vi "Transfer_Curve.vi"(0 "File Path":path=path "C:/DATA/raj/transferdump.txt.txt", 1 "V_G Start":dbl=-0.7 format="%#.3g", 3 "V_G Finish":dbl=0.4 format="%#.3g", 4 "V_G Step Size":dbl=0.05 format="%#.3g", 5 "Preread delay (ms)":dbl=10000.0 format="%.2f", 7 "Delay between \naverages (ms)":dbl=200.0 format="%#.3f", 8 "Keithley 237 GPIB address":string="17", 9 "Software Averages":i16=5, 12 "VISA resource name":refnum<visa-resource-name>="GPIB0::24::INSTR", 13 "First bias settle (ms)":dbl=60000.0 format="%#.2f", 15 "Current Compliance\nLimit (A) Ke2400":dbl=1.0 format="%#.3e", 18 "Dimensions":T1(ring), 24 "Voltage Compliance Limit 237 (V)":dbl=10.0 format="%#.3f", 25 "Current Compliance\nLimit 237 (A)":dbl=0.1 format="%#.3f", 27 "V_DS":dbl=-0.6 format="%#_13g") -> ()   [LabVIEW 2018]
uses:
  <vilib>/Utility/file.llb/Write Delimited Spreadsheet (string).vi
  Instance           1 16Saved   JV curve .vi
  <userlib>/KE237.LLB/Keith 237 Operate/Standby.vi
  <instrlib>/Keithley 24XX/Public/Data/Read (Single Point).vi
  <vilib>/Analysis/NI_AALBase.lvlib
  <instrlib>/Keithley 24XX/Keithley 24XX.lvlib
panel:
  in  "Quick Burn In?":bool
  out "timer":dbl format="%#_6f"
  out "Keithley 2400":cluster{dbl[], dbl[]}(graph)={[-2.0, -1.9, -1.8, -1.7, -1.6, -1.5], [-6.6965744e-11, -6.7804984e-11, -6.685451799999999e-11, -6.6450076e-11, -6.5125542e-11, -6.7339852e-11]}
  out "I_G (A)":dbl=-6.642986e-11 format="%.2e"
  in  "Autozero?":u16(ring) items=["On", "Off", "Once"]
  in  "Measurement Speed (1 PLC)":dbl=1.0 format="%.2g"
  in  "Manual Range (Max I)":dbl=1.0
  in  "Enable Meas Auto Range":bool=TRUE
  in  "Source Mode":u16(ring) items=["Voltage", "Current"]
  in  "Return Sweep?":bool=TRUE
  out "I_DS":dbl=-1.38e-12 format="%.2e"
  out "Outputfile":path=path "C:/DATA/Mark Ziffer/test10"
  in  "Abort Scan":bool=TRUE
  out "V_G":dbl=-1.5 format="%#.2f"
  out "Keithley 237":cluster{dbl[], dbl[]}(graph)={[-2.0, -1.9, -1.8, -1.7, -1.6, -1.5], [-6.720000000000001e-13, -2.18e-13, -2.7599999999999993e-13, -8.999999999999998e-14, -1.3999999999999998e-13, -1.3800000000000002e-13]}
  # "Transfer Curve\nbased on  EL_photocurrent_JV.vi for controlling 2 Ketthleys\n\n9/2017 MZ"
  # "Software Settings"
  # "Ke237 Settings"
  # "Ke2400 Settings"
  # "Notes for IV Scan\n\n2010.07.06 - add absolute value plotter to look at log-scale current\n2010.01.07 - Modified file headers for distinguihing when imported to Igor Pro - the prefix of each header will be the file name.\n2009.01.15 - I updated the code to run on the VISA driver convention. I also modified the file saving and the option to set the\n                      graph display.\n2008.12.01 - I fixed an issue with calculations of J. It was mis-wired to divide current by wavelength, rather than active area.  BM\n\n=========================\nI added the functionality to calculate the fill factor, rectification ratio, short circuit current density, and open circuit voltage. \nAdditionally, current density (mA/cm^2) is reported in the plot window and column B of the data file, and the current (A) has been \nmoved to column C. Open circuit voltage is linearly interpolated. The max power point (mpp) for calculating fill factor is taken as \nthe data point with the highest I-V product, so this makes it only as accurate as your voltage step size, but should be fine for a decent \ndevice on the 50 mV default step size.\n\nIf you know how to use the previous versions of IV scan, \nmake sure you set these parameters before you scan:\n1) Recftification Ratio Bias - this is the +/- bias value you wish to record a rectification ratio at.\n2) Effective Area - this is the area in cm^2 of the diode mask (photoactive area) when measuring under illumination or the measured \n     area of the electrode overlap when measured in dark (regular active area).\n3) Do you want to record a separate data file for the calculated characteristics? If so, make sure the switch is on.\n\nAs of today, I couldn't figure out how to append the computed characteristics to the I-V file without experiencing formating issues, so\nI opted to just create a separate file if you want to save that info. Feel free to fix this if you know how. Check tab 3 > tab 2 > tab 9 in the\nblock diagram.\n\n2008-04-15\nB MacLeod"
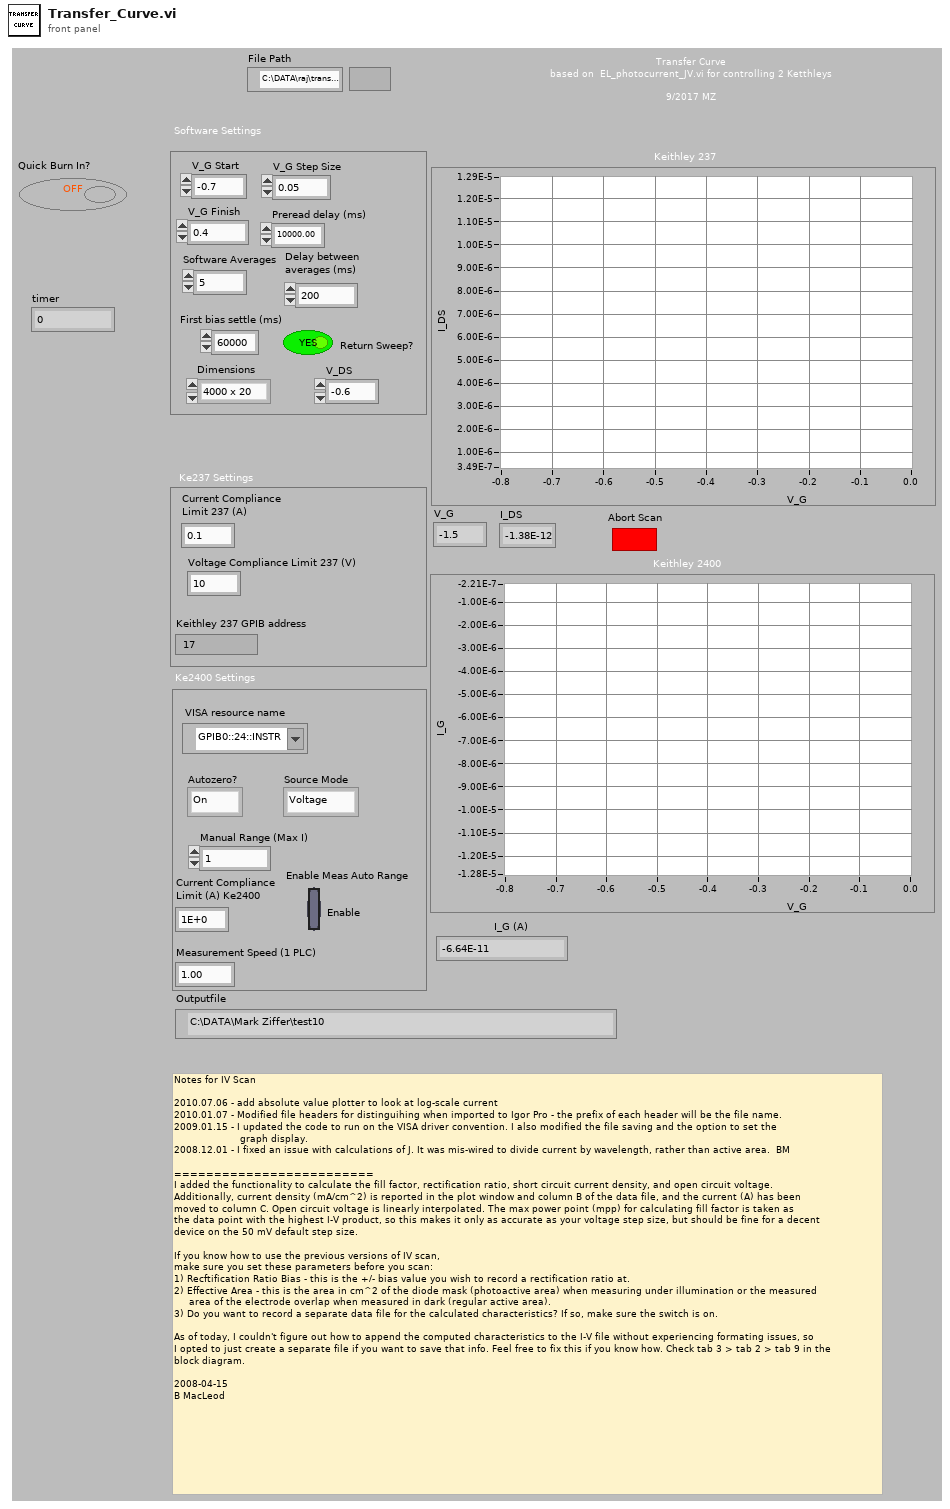
[diagram p1: front panel]
types:
  T1 = enum16{"4000 x 20", "2000 x 20", "1000 x 20", "800 x 20", "400 x 20", "200 x 20", "100 x 20"}
  T2 = cluster{"error":bool, "code":i32, "source":string}
  T3 = cluster{"source value":string, "measure value":string, "delay value (sec)":string, "time value (sec)":string}[]
  T4 = cluster{"source value":dbl, "measure value":dbl, "delay value (sec)":dbl, "time value (sec)":dbl}[]
  T5 = cluster{"[0]":cluster{"source value":dbl, "measure value":dbl, "delay value (sec)":dbl, "time value (sec)":dbl}, "[1]":cluster{"source value":dbl, "measure value":dbl, "delay value (sec)":dbl, "time value (sec)":dbl}, "[2]":cluster{"source value":dbl, "measure value":dbl, "delay value (sec)":dbl, "time value (sec)":dbl}, "[3]":cluster{"source value":dbl, "measure value":dbl, "delay value (sec)":dbl, "time value (sec)":dbl}, "[4]":cluster{"source value":dbl, "measure value":dbl, "delay value (sec)":dbl, "time value (sec)":dbl}, "[5]":cluster{"source value":dbl, "measure value":dbl, "delay value (sec)":dbl, "time value (sec)":dbl}, "[6]":cluster{"source value":dbl, "measure value":dbl, "delay value (sec)":dbl, "time value (sec)":dbl}, "[7]":cluster{"source value":dbl, "measure value":dbl, "delay value (sec)":dbl, "time value (sec)":dbl}, "[8]":cluster{"source value":dbl, "measure value":dbl, "delay value (sec)":dbl, "time value (sec)":dbl}}
  T6 = cluster{"source value":dbl, "measure value":dbl, "delay value (sec)":dbl, "time value (sec)":dbl}
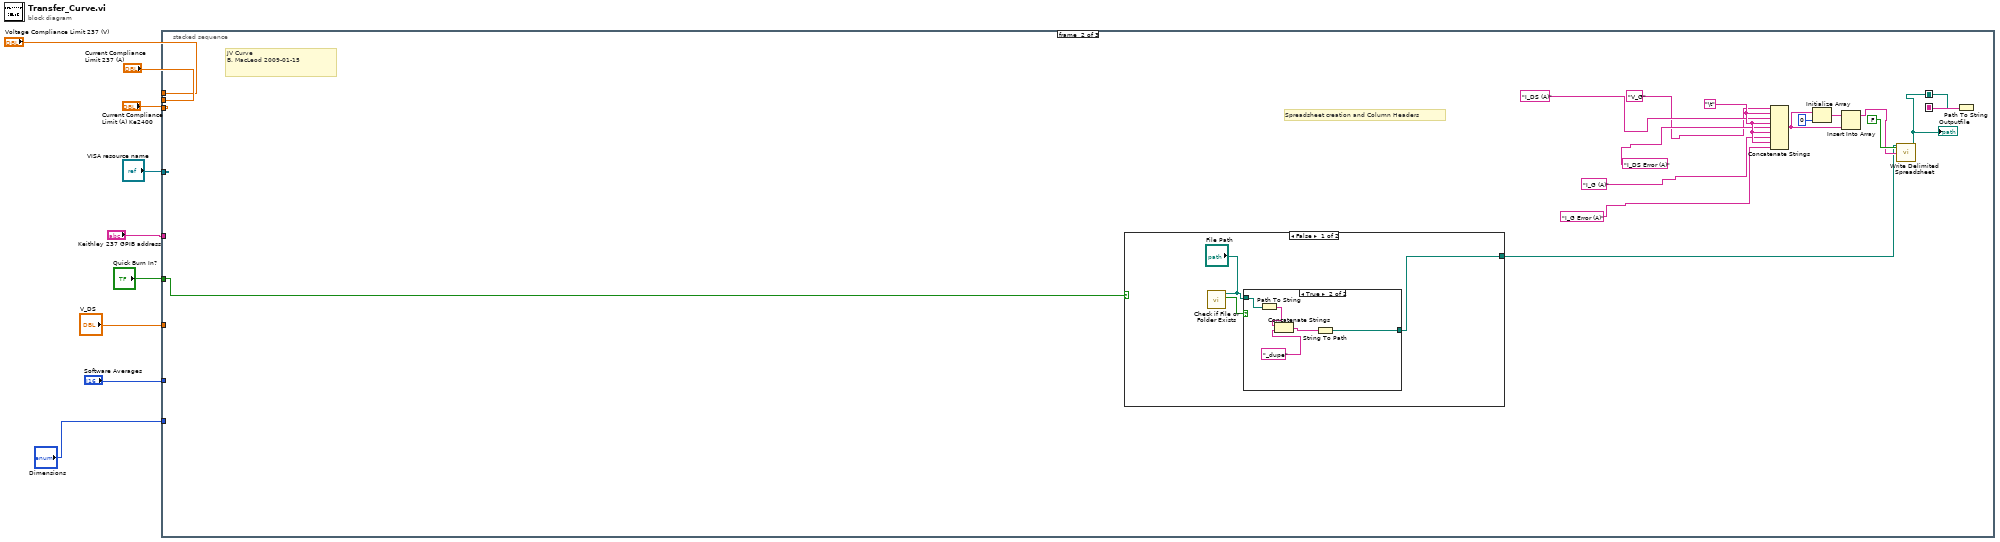
[diagram p0: block diagram]
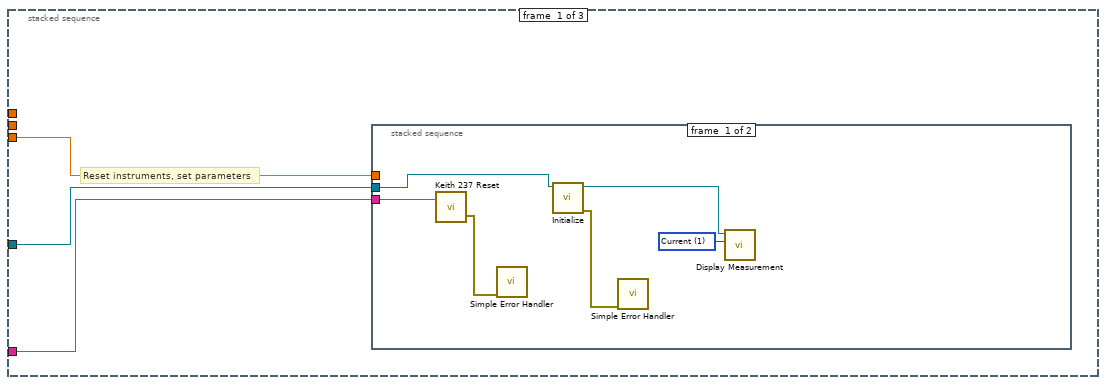
[diagram p2: hidden frame]
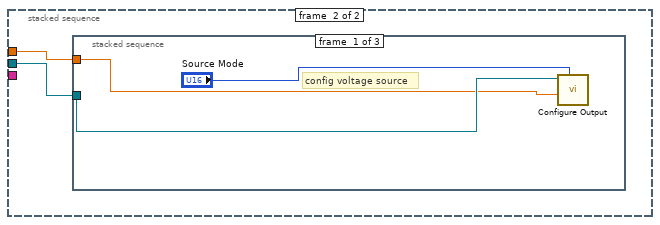
[diagram p3: hidden frame]
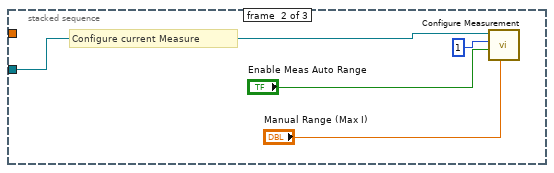
[diagram p4: hidden frame]
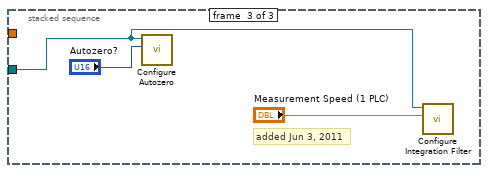
[diagram p5: hidden frame]
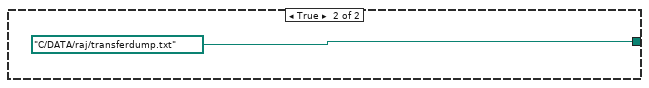
[diagram p7: hidden frame]
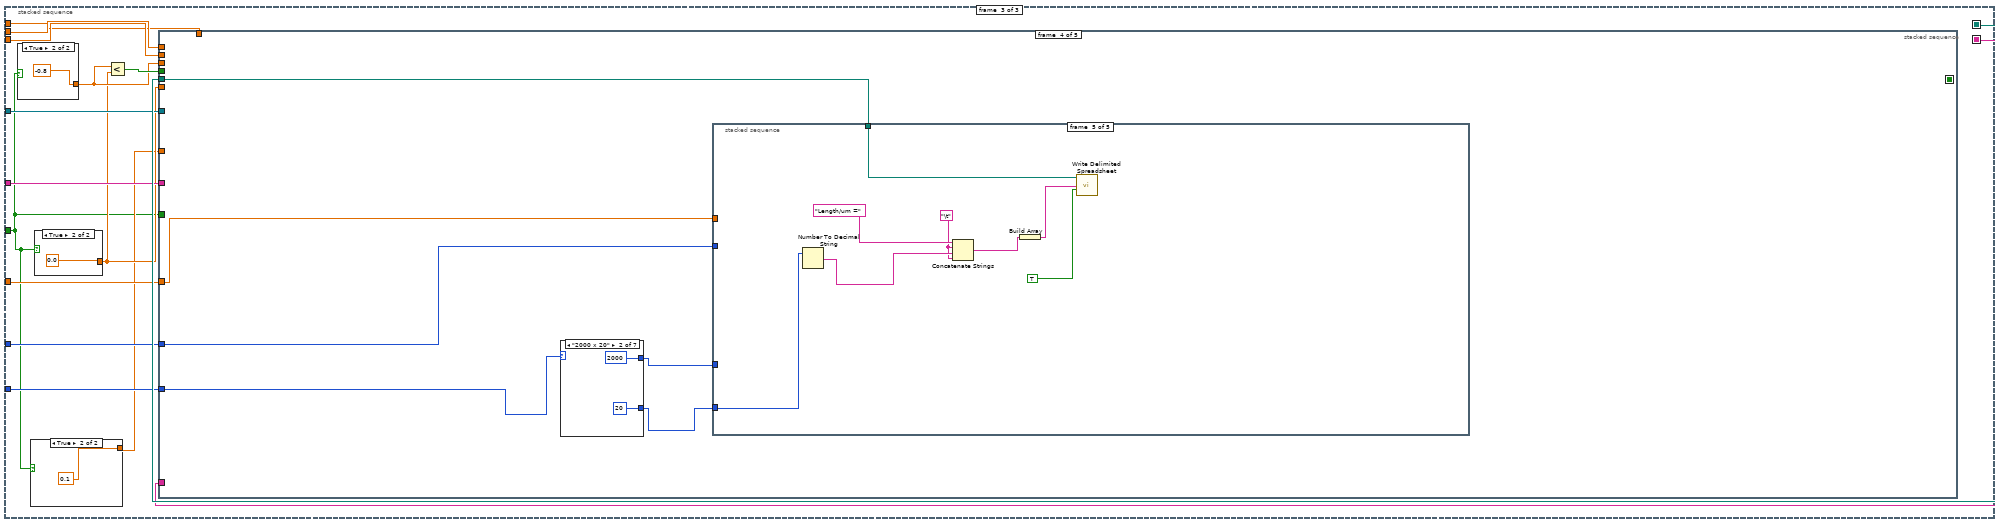
[diagram p8: hidden frame]
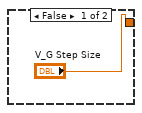
[diagram p9: hidden frame]
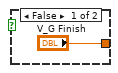
[diagram p10: hidden frame]
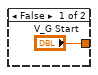
[diagram p11: hidden frame]
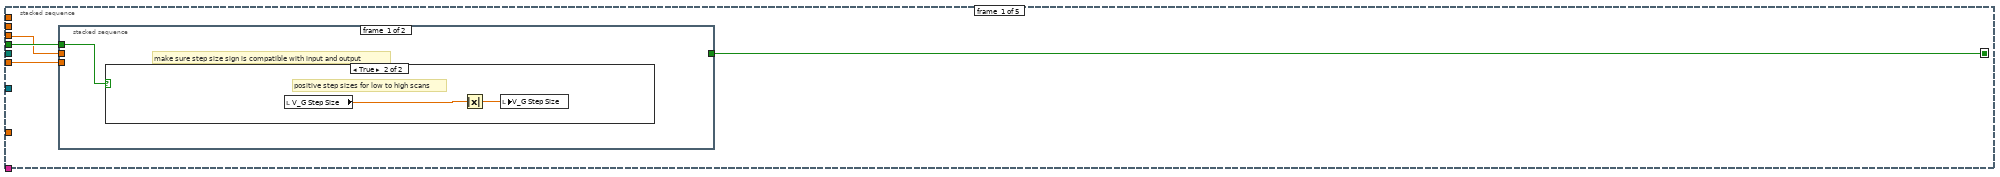
[diagram p12: hidden frame]
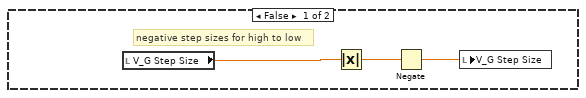
[diagram p13: hidden frame]
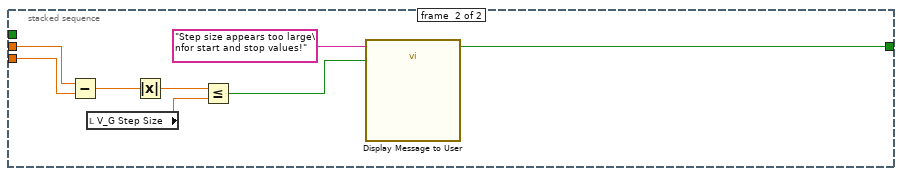
[diagram p14: hidden frame]
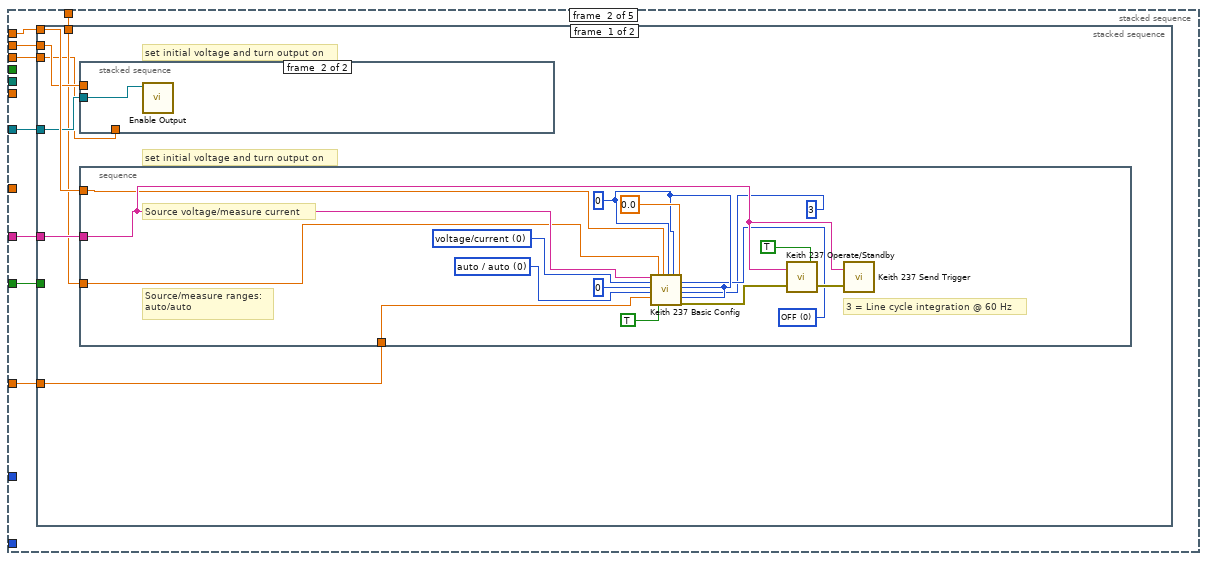
[diagram p15: hidden frame]
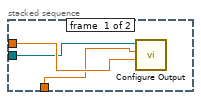
[diagram p16: hidden frame]
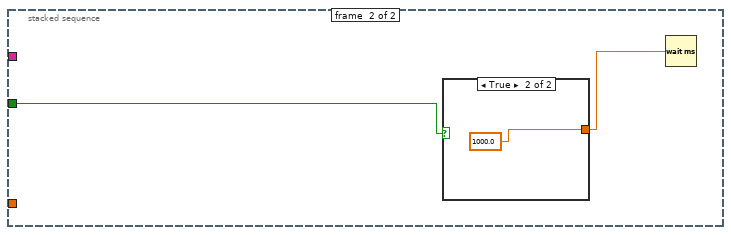
[diagram p17: hidden frame]
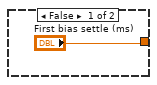
[diagram p18: hidden frame]
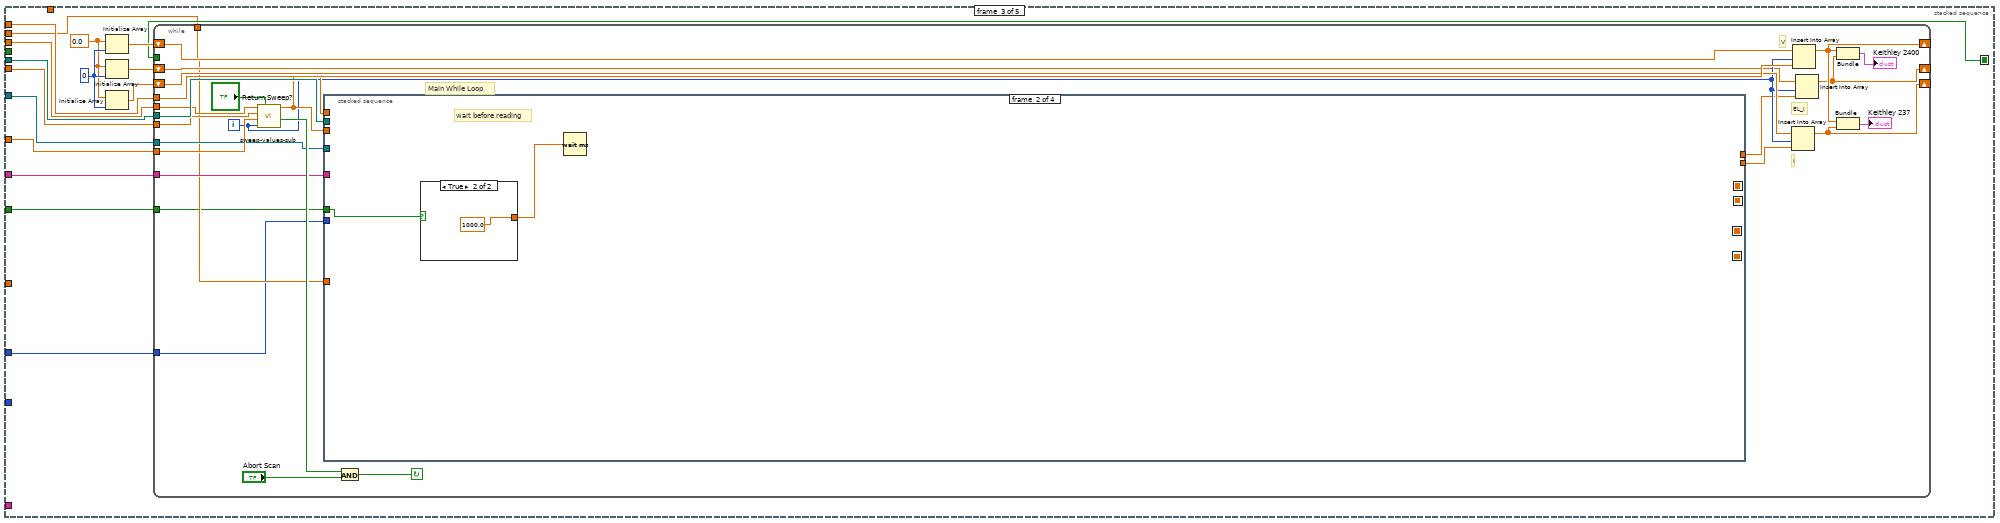
[diagram p19: hidden frame]
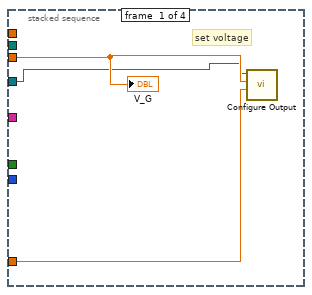
[diagram p20: hidden frame]
diagram:
  # "JV Curve\nB. MacLeod 2009-01-15"
  n1 = stacked-sequence {
    seq-local: [_ w38 _] -> [_ _ w69]
    seq-local: [_ w45 _] -> [_ _ w68]
    tunnel: "Current Compliance\nLimit 237 (A)" -> [_ _ w67]
    tunnel: "Voltage Compliance Limit 237 (V)" -> [_ _ w63]
    tunnel: "Keithley 237 GPIB address" -> [w12 _ w66]
    tunnel: "VISA resource name" -> [w11 _ w65]
    tunnel: "Current Compliance\nLimit (A) Ke2400" -> [w10 _ w64]
    tunnel: "V_DS" -> [_ _ w62]
    tunnel: "Software Averages" -> [_ _ w61]
    tunnel: "Dimensions" -> [_ _ w60]
    tunnel: "Quick Burn In?" -> [_ w31 w56]
    frame #0 {
      # "Reset instruments, set parameters"
      n2 = stacked-sequence {
        tunnel: w12 -> [w17 _]
        tunnel: w11 -> [w16 w20]
        tunnel: w10 -> [_ w19]
        frame #0 {
          w15 = u16 1 items=["Voltage", "Current", "Resistance"] ("Displayed Measurement (0: Voltage)")
          n3 = call <userlib>:"Keith 237 Reset.vi"("GPIB address"=w17) -> ("error out"=w18:T2)  [unwired: 1 in]
          n4 = call <vilib>:"Simple Error Handler.vi"("error in (no error)"=w18) -> ()  [unwired: 1 in, 8 out]
          n5 = call <instrlib>:"Initialize.vi"("VISA resource name"=w16) -> ("error out"=w13:errorcluster, "VISA resource name out"=w14:refnum<visa-resource-name>)  [unwired: 9 in]
          n6 = call <vilib>:"Simple Error Handler.vi"("error in (no error)"=w13) -> ()  [unwired: 1 in, 8 out]
          n7 = call <instrlib>:"Display Measurement.vi"("Displayed Measurement (0: Voltage)"=w15, "VISA resource name"=w14) -> ()  [unwired: 8 in, 2 out]
        }
        frame #1 {
          n8 = stacked-sequence {
            tunnel: w20 -> [w22 w24 w28]
            tunnel: w19 -> [w21 _ _]
            frame #0 {
              # "config voltage source"
              n9 = call <instrlib>:"Configure Output.vi"("Source Mode  (0: Voltage)"="Source Mode", "Compliance  Level (0.1)"=w21, "VISA resource name"=w22) -> ()  [unwired: 3 in, 6 out]
            }
            frame #1 {
              # "Configure current Measure"
              n10 = call <instrlib>:"Configure Measurement.vi"("Manual Range (1.0)"="Manual Range (Max I)", "Enable Auto Range (T:Enable)"="Enable Meas Auto Range", "Function (0: Volts)"=1, "VISA resource name"=w24) -> ()  [unwired: 1 in, 7 out]
            }
            frame #2 {
              # "added Jun 3, 2011"
              n11 = call <instrlib>:"Configure Autozero.vi"("Autozero  (0: On)"="Autozero?", "VISA resource name"=w28) -> ()  [unwired: 1 in, 9 out]
              n12 = call <instrlib>:"Configure Integration Filter.vi"("Measurement Speed (1 PLC)"="Measurement Speed (1 PLC)", "VISA resource name"=w28) -> ()  [unwired: 8 in, 2 out]
            }
          }
        }
      }
    }
    frame #1 {
      w41 = "\t"
      # "Spreadsheet creation and Column Headers"
      n13 = case shown="False" w31 {
        tunnel: [w46 path "C:/DATA/raj/transferdump.txt"] -> w32
        frame False {
          n14 = call <vilib>:"Check if File or Folder Exists.vi"("path"="File Path") -> ("file or folder exists?"=w48:bool)  [unwired: 8 in, 2 out]
          n15 = case shown="True" w48 {
            tunnel: "File Path" -> [w49 w53]
            tunnel: [w49 w50] -> w46
            frame False {
            }
            frame True {
              n16 = Path To String(path=w53) -> (string=w54:string)
              n17 = Concatenate Strings(w54, "_dupe") -> (w51:string)
              n18 = String To Path(string=w51) -> (path=w50:path)
            }
          }
        }
        frame True {
        }
      }
      n19 = Concatenate Strings("V_G", w41, "I_DS (A)", w41, "I_DS Error (A)", w41, "I_G (A)", w41, "I_G Error (A)" ("string")) -> (w43:string)
      n20 = Initialize Array(w43, 0 ("dimension size")) -> (w42:string[])
      n21 = Insert Into Array(array=w42, new element=w43) -> (w39:string[])  [unwired: 1 in]
      n22 = call-poly <vilib>:"Write Delimited Spreadsheet.vi"("file path (dialog if empty)"=w32, "1D data"=w39, "transpose? (no:F)"=FALSE ("append to file? (new file:F)")) -> ("new file path (Not A Path if cancelled)"=w38:path)  [unwired: 11 in, 1 out]
      "Outputfile" <- w38
      n23 = Path To String(path=w38) -> (string=w45:string)
    }
    frame #2 {
      n24 = case shown="True" w56 {
        tunnel: ["V_G Start" -0.8] -> w59
        frame False {
        }
        frame True {
        }
      }
      n25 = case shown="True" w56 {
        tunnel: ["V_G Step Size" 0.1] -> w57
        frame False {
        }
        frame True {
        }
      }
      n26 = case shown="True" w56 {
        tunnel: ["V_G Finish" 0.0] -> w58
        frame False {
        }
        frame True {
        }
      }
      n27 = Less?(x=w59, y=w58) -> (x < y?=w70:bool)
      n28 = stacked-sequence {
        seq-local: [w77 _ _ _ _] -> [_ _ w141 _ _]
        tunnel: w70 -> [w80 _ _ _ _]
        tunnel: w59 -> [w79 w97 w147 _ _]
        tunnel: w58 -> [w78 _ w148 _ _]
        tunnel: w57 -> [_ _ w146 _ _]
        tunnel: w69 -> [_ _ w145 w225 _]
        tunnel: w68 -> [_ _ _ _ _]
        tunnel: w67 -> [_ w102 w142 _ _]
        tunnel: w66 -> [_ w101 w140 _ w281]
        tunnel: w65 -> [_ w99 w139 _ w280]
        tunnel: w64 -> [_ w100 w135 _ _]
        tunnel: w63 -> [_ w98 _ _ _]
        tunnel: w62 -> [_ w96 _ w226 _]
        tunnel: w61 -> [_ _ w134 w224 _]
        tunnel: w60 -> [_ _ _ w223 _]
        tunnel: w56 -> [_ w95 w133 _ _]
        frame #0 {
          n29 = stacked-sequence {
            tunnel: w80 -> [w81 _]
            tunnel: w79 -> [_ w94]
            tunnel: w78 -> [_ w93]
            tunnel: [_ w87] -> w77
            frame #0 {
              # "make sure step size sign is compatible with input and output"
              n30 = case shown="True" w81 {
                frame False {
                  # "negative step sizes for high to low"
                  n31 = local read "V_G Step Size"() -> (w84:dbl)
                  n32 = Absolute Value(x=w84) -> (abs(x)=w83:dbl)
                  n33 = Negate(x=w83) -> (-x=w82:dbl)
                  n34 = local write "V_G Step Size"(w82) -> ()
                }
                frame True {
                  # "positive step sizes for low to high scans"
                  n35 = local read "V_G Step Size"() -> (w86:dbl)
                  n36 = Absolute Value(x=w86) -> (abs(x)=w85:dbl)
                  n37 = local write "V_G Step Size"(w85) -> ()
                }
              }
            }
            frame #1 {
              n38 = Subtract(x=w94, y=w93) -> (x-y=w92:dbl)
              n39 = local read "V_G Step Size"() -> (w90:dbl)
              n40 = Absolute Value(x=w92) -> (abs(x)=w91:dbl)
              n41 = Less Or Equal?(x=w91, y=w90) -> (x <= y?=w88:bool)
              n42 = call "Display Message to User"("Enable"=w88, "Message"="Step size appears too large\nfor start and stop values!") -> ("OK"=w87:bool)  [unwired: 1 in, 8 out]
            }
          }
        }
        frame #1 {
          n43 = stacked-sequence {
            tunnel: w102 -> [w109 _]
            tunnel: w101 -> [w108 _]
            tunnel: w100 -> [w107 _]
            tunnel: w99 -> [w106 _]
            tunnel: w98 -> [w105 _]
            tunnel: w97 -> [w104 _]
            tunnel: w96 -> [w103 _]
            tunnel: w95 -> [_ w130]
            frame #0 {
              # "set initial voltage and turn output on"
              # "set initial voltage and turn output on"
              n44 = stacked-sequence {
                tunnel: w107 -> [w112 _]
                tunnel: w106 -> [w111 w113]
                tunnel: w104 -> [w110 _]
                frame #0 {
                  n45 = call <instrlib>:"Configure Output.vi"("Compliance  Level (0.1)"=w112, "Output Level (0)"=w110, "VISA resource name"=w111) -> ()  [unwired: 3 in, 6 out]
                }
                frame #1 {
                  n46 = call <instrlib>:"Enable Output.vi"("VISA resource name"=w113) -> ()  [unwired: 2 in, 9 out]
                }
              }
              n47 = stacked-sequence {
                tunnel: w109 -> [w117]
                tunnel: w108 -> [w119]
                tunnel: w105 -> [w116]
                tunnel: w103 -> [w114]
                frame #0 {
                  w118 = u16 0 items=["OFF", "ON"] ("default delay (on:1)")
                  w120 = u16 0 items=["auto / auto", "1 nA / 1.1 V", "10 nA / 11 V", "100 nA / 110 V", "0.001 mA / 1100 V", "0.01 mA / 1100 V", "0.1 mA / 1100 V", "1 mA / 1100 V", "10 mA / 1100 V", "100 mA / 1100 V"] ("source range\nI source / V source (auto:0)")
                  w121 = u16 0 items=["voltage/current", "current/voltage"] ("source/measure (V/I:0)")
                  w123 = u16 0
                  # "3 = Line cycle integration @ 60 Hz"
                  # "Source/measure ranges:\nauto/auto"
                  # "Source voltage/measure current"
                  n48 = call <userlib>:"Keith 237 Basic Config.vi"("GPIB address"=w119, "source/measure (V/I:0)"=w121, "function (DC:0)"=u16 0, "source range\nI source / V source (auto:0)"=w120, "source level"=w114, "voltage \ncompliance level"=w116, "1100 V range (disabled:F)"=TRUE, "current \ncompliance level"=w117, "compliance/\nmeasurement range (auto:0)"=w123, "suppression (off:0)"=w123, "DC delay (sec)"=0.0, "default delay (on:1)"=w118, "filter (disabled:0)"=w123, "integration time (medium:1)"=u16 3, "sense (local:0)"=w123) -> ("error out"=w128:T2)  [unwired: 4 in]
                  n49 = call "Keith 237 Operate/Standby.vi"("source"=TRUE, "error in"=w128, "GPIB address"=w119) -> ("error out"=w126:T2)
                  n50 = call <userlib>:"Keith 237 Send Trigger.vi"("GPIB address"=w119, "error in"=w126) -> ()  [unwired: 1 out]
                }
              }
            }
            frame #1 {
              n51 = case shown="True" w130 {
                tunnel: ["First bias settle (ms)" 1000.0] -> w129
                frame False {
                }
                frame True {
                }
              }
              n52 = Wait (ms)(milliseconds to wait=w129) -> ()  [unwired: 1 out]
            }
          }
        }
        frame #2 {
          w138 = 0
          w137 = 0.0
          n53 = Initialize Array(w137, w138) -> (w144:dbl[])
          n54 = Initialize Array(w137, w138) -> (w136:dbl[])
          n55 = Initialize Array(w137, w138) -> (w143:dbl[])
          n56 = while {
            shift-left: w143 -> [w170]
            shift-right: [w158] -> _
            shift-left: w144 -> [w171]
            shift-right: [w161] -> _
            tunnel: w145 -> [w173]
            tunnel: w146 -> [w169]
            tunnel: w147 -> [w168]
            tunnel: w148 -> [w167]
            tunnel: w142 -> [w165]
            tunnel: w141 -> [_]
            shift-right: [w157] -> _
            shift-left: w136 -> [w153]
            tunnel: w140 -> [w156]
            tunnel: w139 -> [w155]
            tunnel: w135 -> [w151]
            tunnel: w134 -> [w150]
            tunnel: w133 -> [w149]
            i -> [w159]
            stop <- w163 continue-if-true
            # "EL_I"
            # "Main While Loop"
            # "V"
            # "I"
            n57 = call "sweep-values-sub.vi"("Forward/Reverse"="Return Sweep?", "Point Number"=w159, "Step Size"=w169, "Sweep Stop"=w167, "Sweep Start"=w168) -> ("Active"=w164:bool, "Output"=w172:dbl)  [unwired: 2 out]
            n58 = stacked-sequence {
              seq-local: [_ _ w190 _] -> [_ _ _ w207]
              seq-local: [_ _ w184 _] -> [_ _ _ w208]
              seq-local: [_ _ w186 _] -> [_ _ _ w206]
              seq-local: [_ _ w185 _] -> [_ _ _ w205]
              tunnel: [_ _ w184 _] -> w160
              tunnel: w172 -> [w177 _ _ w219]
              tunnel: w173 -> [_ _ _ w210]
              tunnel: w165 -> [_ _ _ _]
              tunnel: w156 -> [_ _ w188 _]
              tunnel: w155 -> [w175 _ w187 _]
              tunnel: [_ _ w186 _] -> w154
              tunnel: w151 -> [w176 _ _ _]
              tunnel: w150 -> [_ _ w183 _]
              tunnel: w149 -> [_ w178 _ _]
              frame #0 {
                # "set voltage"
                n59 = call <instrlib>:"Configure Output.vi"("Compliance  Level (0.1)"=w176, "Output Level (0)"=w177, "VISA resource name"=w175) -> ()  [unwired: 3 in, 6 out]
                "V_G" <- w177
              }
              frame #1 {
                # "wait before reading"
                n60 = case shown="True" w178 {
                  tunnel: ["Preread delay (ms)" 1000.0] -> w179
                  frame False {
                  }
                  frame True {
                  }
                }
                n61 = Wait (ms)(milliseconds to wait=w179) -> ()  [unwired: 1 out]
              }
              frame #2 {
                # "I_DS"
                # "I_G"
                # "read values"
                n62 = for {
                  N: w183 -> [_]
                  tunnel: [w194] -> w189 mode=indexing
                  tunnel: w188 -> [w193]
                  tunnel: w187 -> [w192]
                  tunnel: [w191] -> w182 mode=indexing
                  n63 = stacked-sequence {
                    tunnel: [w199 _] -> w194
                    tunnel: w193 -> [w197 _]
                    tunnel: w192 -> [w196 _]
                    tunnel: [w195 _] -> w191
                    frame #0 {
                      n64 = call <userlib>:"Keith 237 Read Measurement.vi"("GPIB address"=w197) -> ("display"=w202:T3)  [unwired: 1 in, 3 out]
                      n65 = call-poly <instrlib>:"Read.vi"("VISA resource name"=w196) -> ("Current"=w195:sgl)  [unwired: 8 in, 6 out]
                      "I_G (A)" <- w195
                      n66 = Fract/Exp String To Number(string=w202) -> (number=w198:T4)  [unwired: 3 in, 1 out]
                      n67 = Array To Cluster(array=w198) -> (cluster=w201:T5)
                      n68 = Unbundle(w201) -> ("[0]"=w200:T6)  [unwired: 8 out]
                      n69 = Unbundle By Name(w200) -> ("measure value"=w199:dbl)  [unwired: 1 out]
                      "I_DS" <- w199
                    }
                    frame #1 {
                      n70 = Wait (ms)(milliseconds to wait="Delay between \naverages (ms)") -> (millisecond timer value=→"timer":u32)
                    }
                  }
                }
                n71 = call <vilib>:"Std Deviation and Variance.vi"("X"=w182) -> ("mean"=w186:dbl, "standard deviation"=w185:dbl)  [unwired: 1 in, 1 out]
                n72 = call <vilib>:"Std Deviation and Variance.vi"("X"=w189) -> ("mean"=w184:dbl, "standard deviation"=w190:dbl)  [unwired: 1 in, 1 out]
              }
              frame #3 {
                w214 = "\t"
                # "I_G"
                # "write data to file"
                # "X"
                n73 = Format Into String(format string="%#f", w219) -> (resulting string=w217:string)  [unwired: 2 in, 1 out]
                n74 = Number To Exponential String(number=w208) -> (E-format string=w220:string)  [unwired: 3 out]
                n75 = Number To Exponential String(number=w207) -> (E-format string=w216:string)  [unwired: 3 out]
                n76 = Number To Exponential String(number=w206) -> (E-format string=w213:string)  [unwired: 3 out]
                n77 = Number To Exponential String(number=w205) -> (E-format string=w212:string)  [unwired: 3 out]
                n78 = Concatenate Strings(w217, w214, w220, w214, w216, w214, w213, w214, w212) -> (w215:string)
                n79 = Build Array(w215) -> (w211:string[])
                n80 = call-poly <vilib>:"Write Delimited Spreadsheet.vi"("file path (dialog if empty)"=w210, "1D data"=w211, "append to file? (new file:F)"=TRUE) -> ()  [unwired: 11 in, 2 out]
              }
            }
            n81 = Compound Arithmetic op=AND(w164, "Abort Scan") -> (w163:bool)
            n82 = Insert Into Array(array=w170, index=w159, new element=w160) -> (w158:dbl[])
            n83 = Insert Into Array(array=w171, index=w159, new element=w172) -> (w161:dbl[])
            n84 = Insert Into Array(array=w153, index=w159, new element=w154) -> (w157:dbl[])
            n85 = Bundle(w161, w157) -> (→"Keithley 2400":cluster{dbl[], dbl[]})  [unwired: 1 out]
            n86 = Bundle(w161, w158) -> (→"Keithley 237":cluster{dbl[], dbl[]})  [unwired: 1 out]
          }
        }
        frame #3 {
          n87 = case shown="\"2000 x 20\"" w223 {
            tunnel: [4000 2000 1000 800 400 200 100] -> w222
            tunnel: [20 20 20 20 20 20 20] -> w221
            frame "4000 x 20", Default {
            }
            frame "2000 x 20" {
            }
            frame "1000 x 20" {
            }
            frame "800 x 20" {
            }
            frame "400 x 20" {
            }
            frame "200 x 20" {
            }
            frame "100 x 20" {
            }
          }
          n88 = stacked-sequence {
            tunnel: w226 -> [_ w252 _ _ _]
            tunnel: w225 -> [w241 w250 w256 w271 w273]
            tunnel: w224 -> [_ _ w258 _ _]
            tunnel: w222 -> [_ _ _ w266 _]
            tunnel: w221 -> [_ _ _ _ w272]
            frame #0 {
              w246 = ""
              w245 = "\t"
              n89 = Concatenate Strings(w246, w245, w246, w245) -> (w242:string)
              n90 = Build Array(w242) -> (w244:string[])
              n91 = call-poly <vilib>:"Write Delimited Spreadsheet.vi"("file path (dialog if empty)"=w241, "1D data"=w244, "append to file? (new file:F)"=TRUE) -> ()  [unwired: 11 in, 2 out]
            }
            frame #1 {
              w253 = "\t"
              n92 = Number To Fractional String(number=w252, precision (6)=3) -> (F-format string=w251:string)  [unwired: 2 in]
              n93 = Concatenate Strings("V_DS = ", w253, w251, w253) -> (w254:string)
              n94 = Build Array(w254) -> (w249:string[])
              n95 = call-poly <vilib>:"Write Delimited Spreadsheet.vi"("file path (dialog if empty)"=w250, "1D data"=w249, "append to file? (new file:F)"=TRUE) -> ()  [unwired: 11 in, 2 out]
            }
            frame #2 {
              w261 = "\t"
              n96 = Number To Decimal String(number=w258) -> (decimal integer string=w257:string)  [unwired: 1 in]
              n97 = Concatenate Strings("Number of Averages = ", w261, w257, w261) -> (w262:string)
              n98 = Build Array(w262) -> (w260:string[])
              n99 = call-poly <vilib>:"Write Delimited Spreadsheet.vi"("file path (dialog if empty)"=w256, "1D data"=w260, "append to file? (new file:F)"=TRUE) -> ()  [unwired: 11 in, 2 out]
            }
            frame #3 {
              w268 = "\t"
              n100 = Number To Decimal String(number=w266) -> (decimal integer string=w267:string)  [unwired: 1 in]
              n101 = Concatenate Strings("Width/um =", w268, w267, w268) -> (w265:string)
              n102 = Build Array(w265) -> (w264:string[])
              n103 = call-poly <vilib>:"Write Delimited Spreadsheet.vi"("file path (dialog if empty)"=w271, "1D data"=w264, "append to file? (new file:F)"=TRUE) -> ()  [unwired: 11 in, 2 out]
            }
            frame #4 {
              w274 = "\t"
              n104 = Number To Decimal String(number=w272) -> (decimal integer string=w277:string)  [unwired: 1 in]
              n105 = Concatenate Strings("Length/um =", w274, w277, w274) -> (w278:string)
              n106 = Build Array(w278) -> (w279:string[])
              n107 = call-poly <vilib>:"Write Delimited Spreadsheet.vi"("file path (dialog if empty)"=w273, "1D data"=w279, "append to file? (new file:F)"=TRUE) -> ()  [unwired: 11 in, 2 out]
            }
          }
        }
        frame #4 {
          # "reset instrument at end of sweep"
          n108 = call <instrlib>:"Reset.vi"("VISA resource name"=w280) -> ()  [unwired: 9 in, 2 out]
          n109 = call <userlib>:"Keith 237 Reset.vi"("GPIB address"=w281) -> ()  [unwired: 1 in, 1 out]
        }
      }
    }
  }
